vi "stable current error.vi"(0 "Stable Current 2":dbl, 1 "Stable Current 1":dbl, 2 "Tails":dbl, 4 "deadtime":dbl) -> (5 "Delta stable current value":dbl)   [LabVIEW 2016]
doc: "This vi caluculates and returns the stable current internal error."
panel:
  out "Tails error":dbl
  out "dead time error":dbl
  out "Current error":dbl
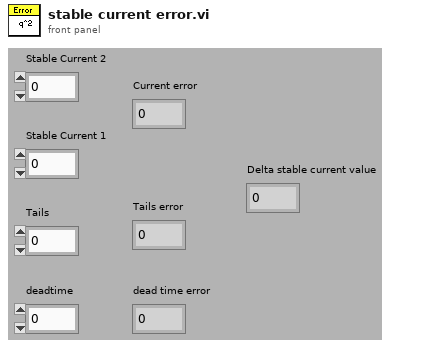
[diagram p1: front panel]
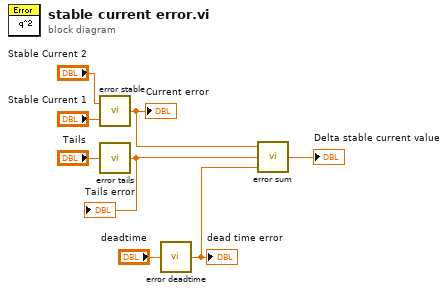
[diagram p0: block diagram]
diagram:
  n1 = call "error stable.vi"("Stable Current 1"="Stable Current 1", "Stable Current 2"="Stable Current 2") -> ("Current error"=w4:dbl)
  "Current error" <- w4
  n2 = call "error tails.vi"("Tails"="Tails") -> ("Tails error"=w3:dbl)
  "Tails error" <- w3
  n3 = call "error deadtime.vi"("deadtime"="deadtime") -> ("dead time error"=w2:dbl)
  "dead time error" <- w2
  n4 = call "error sum.vi"("dead time error"=w2, "Tails error"=w3, "Current error"=w4) -> ("Delta stable current value"=→"Delta stable current value":dbl)
